vi "simplegit.DailyBranchPrefix.vi"() -> (3 "value":string)   [LabVIEW 2017]
uses:
  <resource>/dialog/lvconfig.llb/LV Config Read String.vi
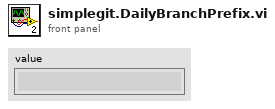
[diagram p1: front panel]
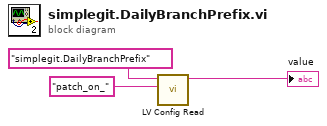
[diagram p0: block diagram]
diagram:
  n1 = call-poly <resource>:"LV Config Read.vi"("default value"="patch_on_" ("DailyBranch Prefix"), "key"="simplegit.DailyBranchPrefix") -> ("value"=→"value":string)  [unwired: 3 in, 2 out]
